vi "Set Voltage and Current.vi"(7 "Wait?":bool, 8 "error in (no error)":errorcluster, 9 "Current Limit":dbl, 10 "Voltage Limit":dbl, 11 "Magna Power in":refnum<class "Magna Power.lvclass">) -> (0 "error out":errorcluster, 3 "Magna Power out":refnum<class "Magna Power.lvclass">)   [LabVIEW 2012, in "Magna Power.lvclass"]
uses:
  Magna Power.lvclass
  Magna Power.lvclass/Magna Power.ctl
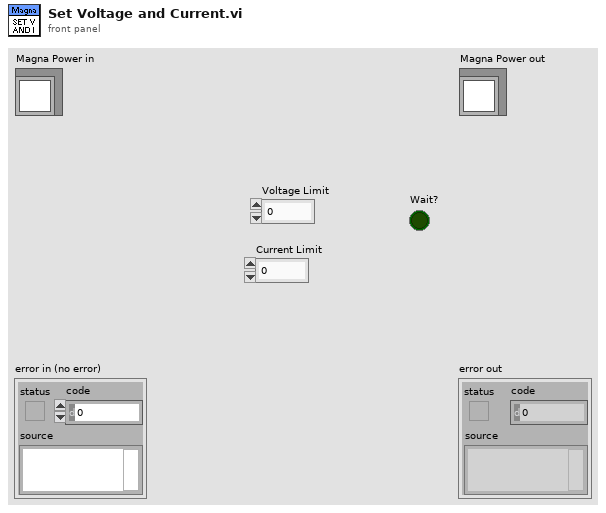
[diagram p1: front panel]
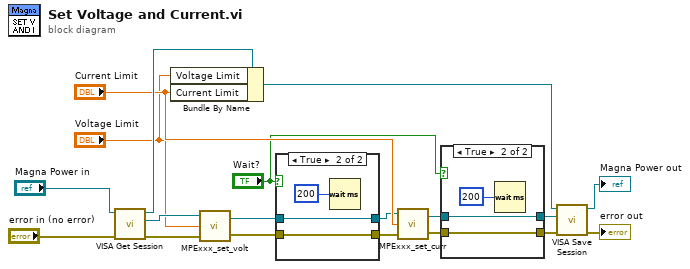
[diagram p0: block diagram]
diagram:
  n1 = call-dynamic "VISA Get Session.vi"("error in (no error)"="error in (no error)", "Instrument.lvclass in"="Magna Power in") -> ("error out"=w17:errorcluster, "VISA Resource Name"=w16:refnum<visa-resource-name>, "Instrument.lvclass out"=w18:refnum<class "Magna Power.lvclass">)  [unwired: 6 in, 1 out]
  n2 = Bundle By Name(cluster=w18, "Voltage Limit"="Voltage Limit", "Current Limit"="Current Limit") -> (w19:refnum<class "Magna Power.lvclass">)
  n3 = call "MPExxx_set_volt.vi"("error in (no error)"=w17, "Set Voltage"="Voltage Limit", "VISA session"=w16) -> ("error out"=w6:errorcluster, "dup VISA session"=w7:refnum<visa-resource-name>)
  n4 = case shown="True" "Wait?" {
    tunnel: [w21 w24] -> w8
    tunnel: w7 -> [w21 w24]
    tunnel: w6 -> [w20 w23]
    tunnel: [w20 w23] -> w9
    frame False {
    }
    frame True {
      n5 = Wait (ms)(milliseconds to wait=u32 200) -> ()  [unwired: 1 out]
    }
  }
  n6 = call "MPExxx_set_curr.vi"("error in (no error)"=w9, "Set Current"="Current Limit", "VISA session"=w8) -> ("error out"=w5:errorcluster, "dup VISA session"=w4:refnum<visa-resource-name>)
  n7 = case shown="True" "Wait?" {
    tunnel: [w26 w29] -> w3
    tunnel: w4 -> [w26 w29]
    tunnel: w5 -> [w25 w28]
    tunnel: [w25 w28] -> w2
    frame False {
    }
    frame True {
      n8 = Wait (ms)(milliseconds to wait=u32 200) -> ()  [unwired: 1 out]
    }
  }
  n9 = call-dynamic "VISA Save Session.vi"("error in (no error)"=w2, "VISA Resource Name"=w3, "Instrument.lvclass in"=w19) -> ("error out"=→"error out":errorcluster, "Instrument.lvclass out"=→"Magna Power out":refnum<class "Magna Power.lvclass">)  [unwired: 7 in]
